vi "Strip Description.vi"(7 "Config":refnum<class "TAF Proj Config.lvclass">, 11 "Description in":string) -> (3 "Description out":string)   [LabVIEW 2021, in "TAF Proj Document Type.lvlib" / "Project Parser.lvlib"]
uses:
  <vilib>/Wovalab/AntiDoc/Document Type/Add-ons/LabVIEW TAF Project/Project Parser/Project Parser.lvlib
  <vilib>/Wovalab/AntiDoc/Document Type/Add-ons/LabVIEW TAF Project/TAF Proj Config/TAF Proj Config.lvclass
  <vilib>/Wovalab/AntiDoc/Document Type/Add-ons/LabVIEW TAF Project/TAF Proj Config/TAF Proj Config.lvclass/TAF Proj Config.ctl
  <vilib>/Wovalab/AntiDoc/Document Type/Add-ons/LabVIEW TAF Project/TAF Proj Config/Read Description Strip Tokens.vi
  <vilib>/regexp/Match Regular Expression.xnode
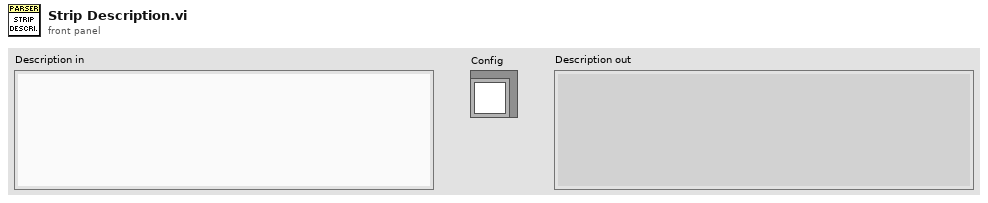
[diagram p1: front panel]
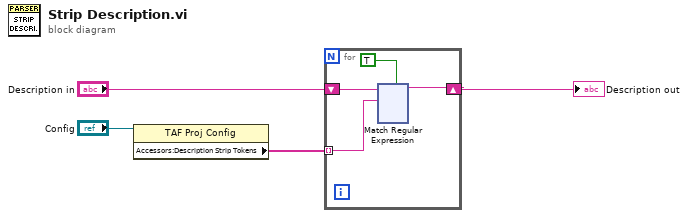
[diagram p0: block diagram]
diagram:
  n1 = property class="TAF Proj Config"(reference="Config") -> ("Accessors:Description Strip Tokens"=w1:string[])  [unwired: 1 in, 2 out]
  n2 = for {
    shift-right: [w7] -> w3
    shift-left: "Description in" -> [w8]
    tunnel: w1 -> [w5] mode=indexing
    n3 = xnode "Match Regular Expression"("input string"=w8, "regular expression"=w5, "multiline? (F)"=TRUE) -> ("before match"=w7:string)  [unwired: 3 in, 4 out]
  }
  "Description out" <- w3
